vi "myRIO_BRig_RT_dataExp_Tcycle_Wrong.vi"() -> (2 "output_Tcycle_Wrong":i32)   [LabVIEW 2014]
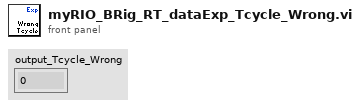
[diagram p1: front panel]
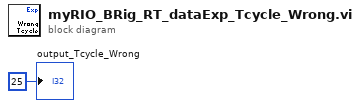
[diagram p0: block diagram]
diagram:
  "output_Tcycle_Wrong" <- 25 ("output_iBlock")
